vi "FRCts20_WebMethods_Comment_POST.vi"(7 "httpRequestID":u32, 11 "request":string) -> ()   [LabVIEW 2013, in "FRCts20_WebMethods.lvlib"]
doc: "<B>POST</B> a new comment resource\n\n<B>Required XML Data : </B>\n<Note>\n <Text><B>string</B></Text>\n <Author><B>string</B></Author>\n</Note>\n\n<B>Required HTML Form Data : </B>\nAuthor: <B>string</B>\nText: <B>string</B>\n\nhttp://<server address>:<port>/FRCts/request/<B>request</B>/comment"
uses:
  FRCts20_WebMethods.lvlib
  <vilib>/wsapi/NI_WebServices.lvlib
  Backend/source/VI Source/FRCts20_Backend_API/FRCts20_Backend_API.lvlib
  Backend/source/VI Source/FRCts20_Backend_API/FRCts20_Backend_API_Note.ctl
  Backend/source/VI Source/FRCts20_Backend_API/FRCts20_Backend_API_Command_Note.ctl
  FRCts20_WebMethods_ReadData_Request.vi
  Backend/source/VI Source/FRCts20_Backend_API/FRCts20_Backend_API_Application.vi
  FRCts20_WebMethods_Redirect_Request.vi
panel:
  in  "query":string
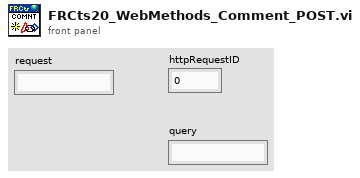
[diagram p1: front panel]
types:
  T1 = typedef "FRCts20_Backend_API.lvlib/FRCts20_Backend_API_Note.ctl" = cluster{"Note Index":u32, "Request Index":u32, "Author":string, "Time Entered":timestamp, "Text":string, "Solution":bool, "APIReturn":string}
  T2 = typedef "FRCts20_Backend_API.lvlib/FRCts20_Backend_API_Command_Note.ctl" = string
  T3 = typedef "FRCts20_WebMethods.lvlib/FRCts20_WebMethods_ctl_request.ctl" = cluster{"Event":string, "Description":string, "Status":T4, "Open Date":string, "Last Update":string, "Close Date":string, "UniqueId":i32, "Team":cluster{"Team Nickname":string, "Team Number ":i32, "UniqueId":i32}, "Comments":cluster{"Request Number":dbl, "Text":string, "Author":string, "IsSolution":bool, "Team":cluster{"Team Nickname":string, "Team Identifier ":dbl}, "UniqueId":i32}[]}
  T4 = typedef "FRCts20_Backend_API.lvlib/FRCts20_Backend_API_Status.ctl" = enum16{"Open", "In Work", "Closed"}
  T5 = typedef "FRCts20_Backend_API.lvlib/FRCts20_Backend_API_Application.ctl" = cluster{"Revision":string, "APIReturn":string}
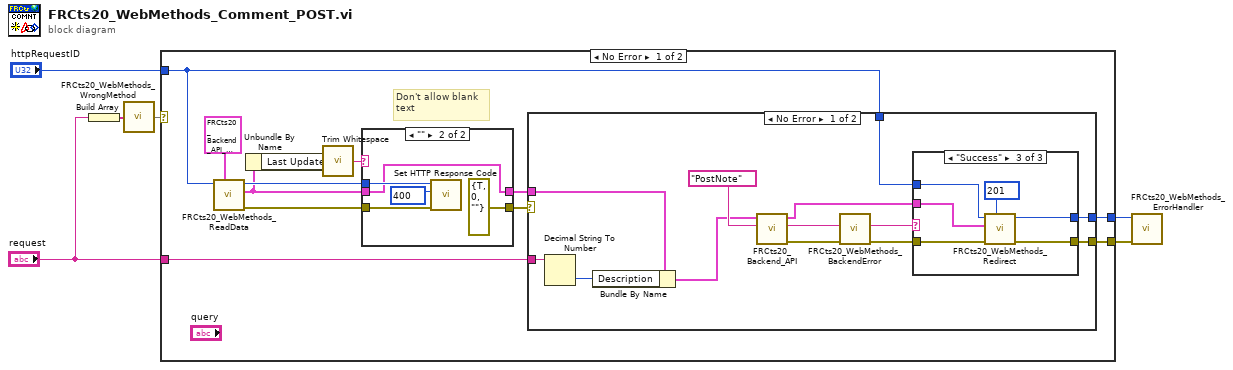
[diagram p0: block diagram]
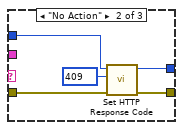
[diagram p4: hidden frame]
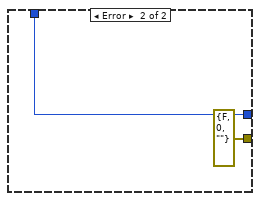
[diagram p5: hidden frame]
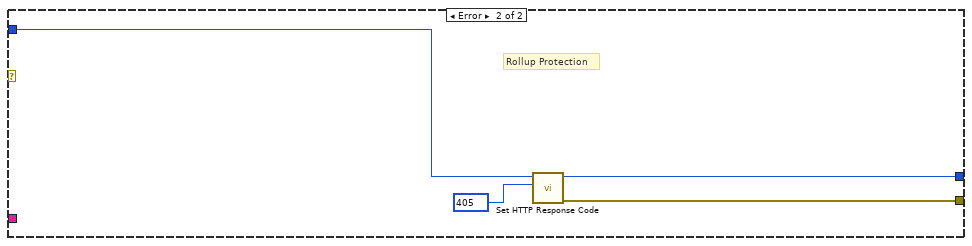
[diagram p6: hidden frame]
diagram:
  n1 = Build Array("request") -> (w5:string[])
  n2 = call "FRCts20_WebMethods_WrongMethod.vi"(4:w5) -> (1:w6)  [unwired: 3 in, 1 out]
  n3 = case shown="No Error" w6 {
    tunnel: "httpRequestID" -> [w14 w57]
    tunnel: [w15 w55] -> w2
    tunnel: [w16 w54] -> w3
    tunnel: "request" -> [w17 _]
    frame No Error {
      # "Don't allow blank\ntext"
      n4 = call-poly "FRCts20_WebMethods_ReadData.vi"(7:T1 {"Note Index"=0, "Request Index"=0, "Author"="", "Time Entered"=timestamp(0 s since 1904-01-01), "Text"="", "Solution"=FALSE, "APIReturn"=""} ("Note"), "httpRequestID"=w14) -> ("error out"=w10:errorcluster, "Request 2"=w7:T3, "httpRequestID out"=w9:u32)  [unwired: 7 in]
      n5 = Unbundle By Name(w7) -> ("Last Update"=w12:string)
      n6 = call <vilib>:"Trim Whitespace.vi"("string"=w12) -> ("trimmed string"=w13:string)  [unwired: 1 in]
      n7 = case shown="\"\"" w13 {
        tunnel: [w20 errorcluster {"status"=TRUE, "code"=0, "source"=""} ("error out")] -> w11
        tunnel: w10 -> [w20 w22]
        tunnel: w9 -> [_ w23]
        tunnel: w7 -> [w19 w21]
        tunnel: [w19 w21] -> w8
        frame Default {
        }
        frame "" {
          w25 = 400 items=["100"=100, "101"=101, "200"=200, "201"=201, "202"=202, "203"=203, "204"=204, "205"=205, "206"=206, "300"=300, "301"=301, "302"=302, "303"=303, "304"=304, "305"=305, "306"=306, "307"=307, "400"=400, "401"=401, "402"=402, "403"=403, "404"=404, "405"=405, "406"=406, "407"=407, "408"=408, "409"=409, "410"=410, "411"=411, "412"=412, "413"=413, "414"=414, "415"=415, "416"=416, "417"=417, "500"=500, "501"=501, "502"=502, "503"=503, "504"=504, "505"=505] ("response code (200)")
          n8 = call <vilib>:"Set HTTP Response Code.vi"("error in (no error)"=w22, "response code (200)"=w25, "httpRequestID"=w23) -> ()  [unwired: 7 in, 2 out]
        }
      }
      n9 = case shown="No Error" w11 {
        tunnel: w17 -> [w38 _]
        tunnel: [w36 errorcluster {"status"=FALSE, "code"=0, "source"=""} ("error out")] -> w16
        tunnel: [w35 w53] -> w15
        tunnel: w14 -> [w29 w53]
        tunnel: w8 -> [w26 _]
        frame No Error {
          n10 = Decimal String To Number(string=w38) -> (number=w37:i32)  [unwired: 2 in, 1 out]
          n11 = Bundle By Name(cluster=w26, "Description"=w37) -> (w27:T3)
          n12 = call-poly "FRCts20_Backend_API.vi"("Command"=T2 "PostNote", 11:w27) -> ("error out"=w32:errorcluster, "Status"=w31:string, "Application"=w34:T5)  [unwired: 7 in]
          n13 = call "FRCts20_WebMethods_BackendError.vi"("error in (no error)"=w32, "Status"=w31) -> ("error out"=w33:errorcluster, "Status out"=w30:string)  [unwired: 8 in]
          n14 = case shown="\"Success\"" w30 {
            tunnel: [w40 w45 w51] -> w36
            tunnel: [w39 w44 w50] -> w35
            tunnel: w34 -> [_ _ w49]
            tunnel: w33 -> [w40 w43 w48]
            tunnel: w29 -> [w39 w42 w47]
            frame "Backend Error", Default {
            }
            frame "No Action" {
              w41 = 409 items=["100"=100, "101"=101, "200"=200, "201"=201, "202"=202, "203"=203, "204"=204, "205"=205, "206"=206, "300"=300, "301"=301, "302"=302, "303"=303, "304"=304, "305"=305, "306"=306, "307"=307, "400"=400, "401"=401, "402"=402, "403"=403, "404"=404, "405"=405, "406"=406, "407"=407, "408"=408, "409"=409, "410"=410, "411"=411, "412"=412, "413"=413, "414"=414, "415"=415, "416"=416, "417"=417, "500"=500, "501"=501, "502"=502, "503"=503, "504"=504, "505"=505] ("response code (200)")
              n15 = call <vilib>:"Set HTTP Response Code.vi"("error in (no error)"=w43, "response code (200)"=w41, "httpRequestID"=w42) -> ("error out"=w45:errorcluster, "httpRequestID out"=w44:u32)  [unwired: 7 in]
            }
            frame "Success" {
              w46 = 201 items=["100"=100, "101"=101, "200"=200, "201"=201, "202"=202, "203"=203, "204"=204, "205"=205, "206"=206, "300"=300, "301"=301, "302"=302, "303"=303, "304"=304, "305"=305, "306"=306, "307"=307, "400"=400, "401"=401, "402"=402, "403"=403, "404"=404, "405"=405, "406"=406, "407"=407, "408"=408, "409"=409, "410"=410, "411"=411, "412"=412, "413"=413, "414"=414, "415"=415, "416"=416, "417"=417, "500"=500, "501"=501, "502"=502, "503"=503, "504"=504, "505"=505] ("response code (200)")
              n16 = call-poly "FRCts20_WebMethods_Redirect.vi"("response code (200)"=w46, "error in (no error)"=w48, "Request"=w49, "httpRequestID"=w47) -> ("error out"=w51:errorcluster, "httpRequestID out"=w50:u32)  [unwired: 6 in]
            }
          }
        }
        frame Error {
        }
      }
    }
    frame Error {
      w56 = 405 items=["100"=100, "101"=101, "200"=200, "201"=201, "202"=202, "203"=203, "204"=204, "205"=205, "206"=206, "300"=300, "301"=301, "302"=302, "303"=303, "304"=304, "305"=305, "306"=306, "307"=307, "400"=400, "401"=401, "402"=402, "403"=403, "404"=404, "405"=405, "406"=406, "407"=407, "408"=408, "409"=409, "410"=410, "411"=411, "412"=412, "413"=413, "414"=414, "415"=415, "416"=416, "417"=417, "500"=500, "501"=501, "502"=502, "503"=503, "504"=504, "505"=505] ("response code (200)")
      # "Rollup Protection"
      n17 = call <vilib>:"Set HTTP Response Code.vi"("response code (200)"=w56, "httpRequestID"=w57) -> ("error out"=w54:errorcluster, "httpRequestID out"=w55:u32)  [unwired: 8 in]
    }
  }
  n18 = call "FRCts20_WebMethods_ErrorHandler.vi"("error in"=w3, "httpRequestID"=w2) -> ()  [unwired: 9 in, 1 out]
